vi "Configure Scale.vi"(7 "Channel Name (1: Channel 1)":i32(ring)=1 items=["Channel 1"=1, "Channel 2"=2, "Channel 3"=3, "Channel 4"=4], 8 "error in (no error)":errorcluster, 9 "Vertical Scale (5 V/div)":dbl=5.0, 10 "Time Scale (0.0001 Sec/div)":dbl=0.0001, 11 "VISA resource name":refnum<visa-resource-name>) -> (0 "error out":errorcluster, 3 "VISA resource name out":refnum<visa-resource-name>)   [LabVIEW 2023, in "Keysight-DSQx3014T.lvlib"]
doc: "Scales the time (horizontal) and vertical axes for the selected analog channel. Use the <b>Configure Channel </b>VI to configure other settings for each analog channel."
uses:
  Keysight-DSQx3014T.lvlib
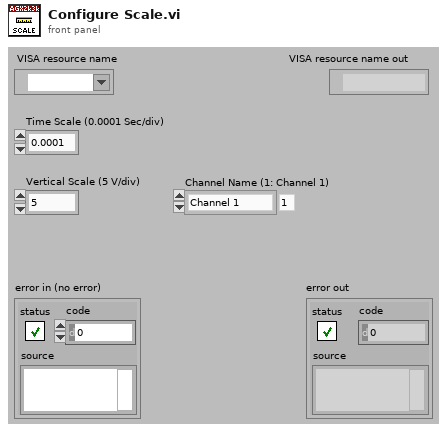
[diagram p1: front panel]
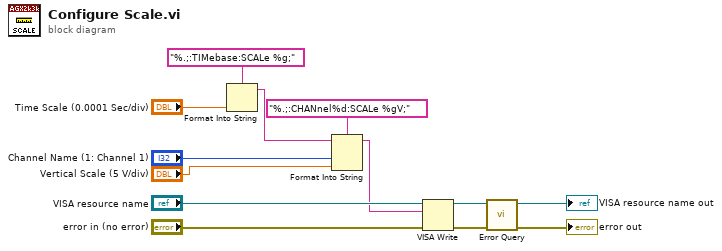
[diagram p0: block diagram]
diagram:
  n1 = Format Into String(format string="%.;:TIMebase:SCALe %g;", "Time Scale (0.0001 Sec/div)") -> (resulting string=w4:string)  [unwired: 2 in, 1 out]
  n2 = Format Into String(format string="%.;:CHANnel%d:SCALe %gV;", initial string=w4, "Channel Name (1: Channel 1)", "Vertical Scale (5 V/div)") -> (resulting string=w3:string)  [unwired: 1 in, 1 out]
  n3 = VISA Write(VISA resource name="VISA resource name", write buffer=w3, error in (no error)="error in (no error)") -> (VISA resource name out=w9:refnum<visa-resource-name>, error out=w8:errorcluster)  [unwired: 1 out]
  n4 = call "Error Query.vi"("error in (no error)"=w8, "VISA resource name"=w9) -> ("error out"=→"error out":errorcluster, "VISA resource name out"=→"VISA resource name out":refnum<visa-resource-name>)  [unwired: 6 in, 2 out]
